vi "parse_dictionary_file.vi"(8 "error_in":errorcluster, 11 "csv_string":string) -> (0 "error_out":errorcluster, 3 "dictionary":T1)   [LabVIEW 2020]
uses:
  Dictionary--Cluster.ctl
  Font -- Cluster.ctl
  Phrase Dictionary Entry -- Cluster.ctl
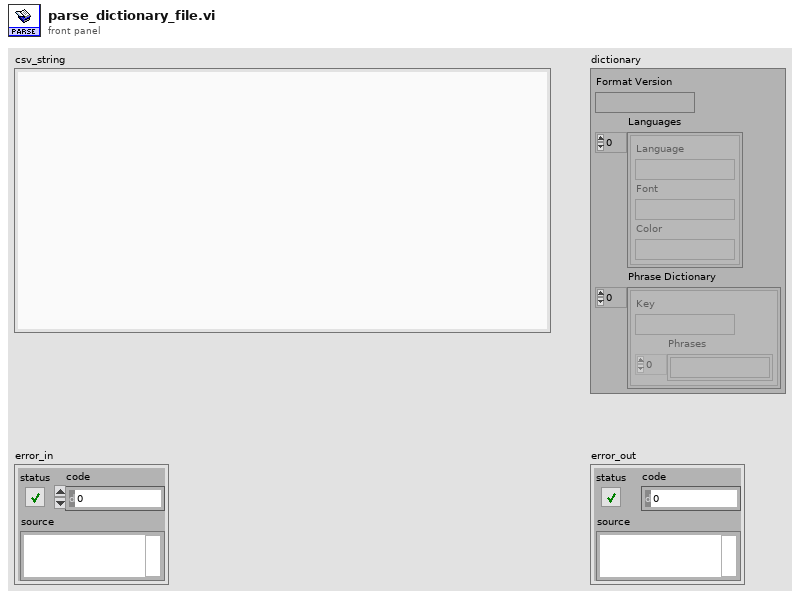
[diagram p1: front panel]
types:
  T1 = typedef "Dictionary--Cluster.ctl" = cluster{"Format Version":string, "Languages":T2[], "Phrase Dictionary":T3[]}
  T2 = typedef "Font -- Cluster.ctl" = cluster{"Language":string, "Font":string, "Color":string}
  T3 = typedef "Phrase Dictionary Entry -- Cluster.ctl" = cluster{"Key":string, "Phrases":string[]}
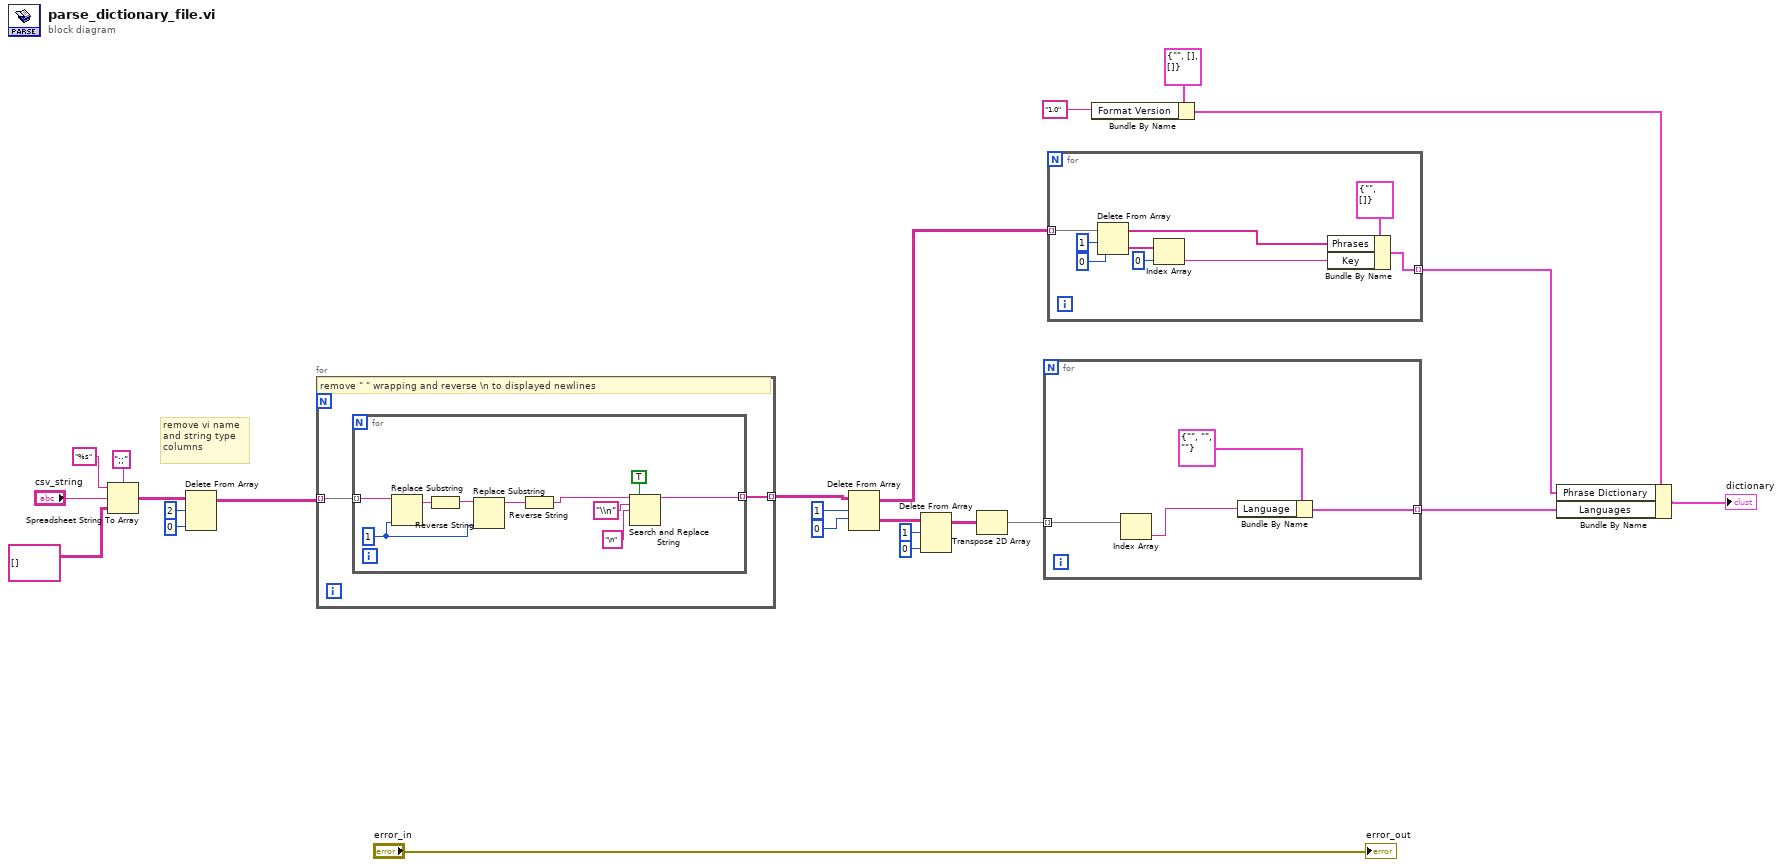
[diagram p0: block diagram]
diagram:
  # "remove vi name\nand string type\ncolumns"
  n1 = Spreadsheet String To Array(delimiter (Tab)=";;", format string="%s", spreadsheet string="csv_string", array type (2D Dbl)=string[][] []) -> (array=w4:string[][])
  n2 = Delete From Array(array=w4, length=2, index (col)=0 ("disabled index (col)")) -> (array with subset deleted=w3:string[][])  [unwired: 1 in, 1 out]
  n3 = for {
    tunnel: w3 -> [w26] mode=indexing
    tunnel: [w25] -> w5 mode=indexing
    # "remove \" \" wrapping and reverse \\n to displayed newlines"
    n4 = for {
      tunnel: w26 -> [w36] mode=indexing
      tunnel: [w27] -> w25 mode=indexing
      w32 = 1 ("length (len. of substring)")
      n5 = Replace Substring(2:w32, 5:w36) -> (1:w35:string)  [unwired: 2 in, 1 out]
      n6 = Reverse String(1:w35) -> (0:w34:string)
      n7 = Replace Substring(2:w32, 5:w34) -> (1:w33:string)  [unwired: 2 in, 1 out]
      n8 = Reverse String(1:w33) -> (0:w28:string)
      n9 = Search and Replace String(replace all?=TRUE ("replace all? (F)"), input string=w28, search string="\\n", replace string="\n" ("replace string (\"\")")) -> (result string=w27:string)  [unwired: 4 in, 3 out]
    }
  }
  n10 = Delete From Array(array=w5, length=1, index (row)=0) -> (deleted portion=w15:string[][], array with subset deleted=w8:string[][])  [unwired: 1 in]
  n11 = Delete From Array(array=w15, length=1, index (col)=0 ("disabled index (col)")) -> (array with subset deleted=w12:string[][])  [unwired: 1 in, 1 out]
  n12 = Transpose 2D Array(2D array=w12) -> (transposed array=w11:string[][])
  n13 = for {
    tunnel: w11 -> [w39] mode=indexing
    tunnel: [w37] -> w9 mode=indexing
    n14 = Index Array(array=w39) -> (element=w38:string)  [unwired: 1 in]
    n15 = Bundle By Name(cluster=T2 {"Language"="", "Font"="", "Color"=""} ("Font"), "Language"=w38) -> (w37:T2)
  }
  n16 = for {
    tunnel: w8 -> [w47] mode=indexing
    tunnel: [w48] -> w7 mode=indexing
    n17 = Delete From Array(array=w47, length=1, index=0) -> (deleted portion=w44:string[], array with subset deleted=w41:string[])
    n18 = Index Array(array=w44, index=0) -> (element=w42:string)
    n19 = Bundle By Name(cluster=T3 {"Key"="", "Phrases"=[]} ("Phrase Dictionary"), "Phrases"=w41, "Key"=w42) -> (w48:T3)
  }
  n20 = Bundle By Name(cluster=T1 {"Format Version"="", "Languages"=[], "Phrase Dictionary"=[]} ("Localization"), "Format Version"="1.0") -> (w10:T1)
  n21 = Bundle By Name(cluster=w10, "Phrase Dictionary"=w7, "Languages"=w9) -> (→"dictionary":T1)
  "error_out" <- "error_in"
